vi "Launch Process.vi"(8 "error in (no error)":errorcluster, 11 "ConfigManager.Text in":refnum<class "ConfigManager.Text.lvclass">) -> (0 "error out":errorcluster, 2 "Process started":bool, 3 "ConfigManager.Text out":refnum<class "ConfigManager.Text.lvclass">)   [LabVIEW 2013, in "CfgManager.Text.lvlib" / "ConfigManager.Text.lvclass"]
uses:
  ConfigManager.Text.lvclass
  ConfigManager.Text.lvclass/ConfigManager.Text.ctl
  Process.vi
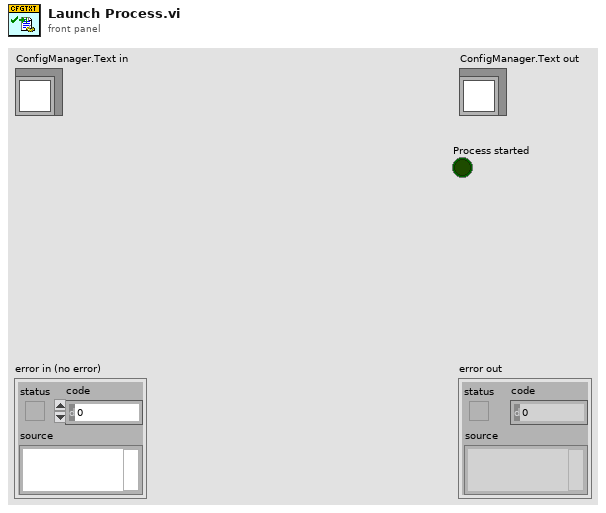
[diagram p1: front panel]
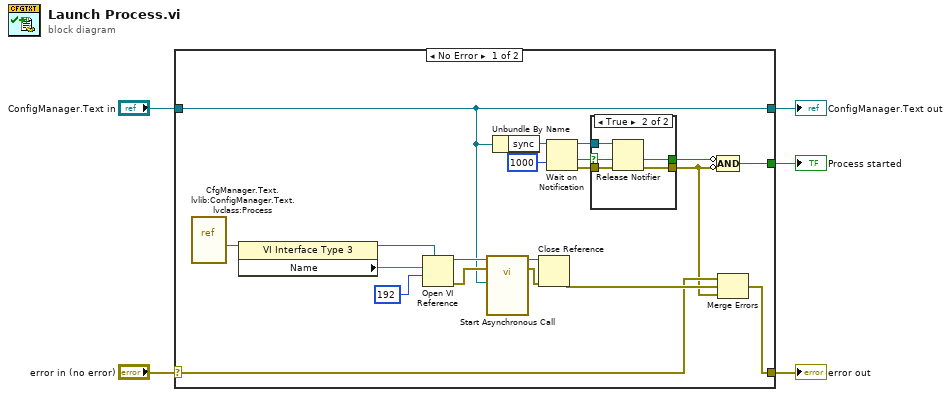
[diagram p0: block diagram]
diagram:
  n1 = case shown="No Error" "error in (no error)" {
    selector: "error in (no error)" -> [w13 w33]
    tunnel: [w12 w33] -> w4
    tunnel: [w17 w32] -> w2
    tunnel: "ConfigManager.Text in" -> [w17 w32]
    tunnel: [w11 _] -> w1
    frame No Error {
      n2 = vi-ref "CfgManager.Text.lvlib:ConfigManager.Text.lvclass:Process.vi"() -> (w25:refnum<vi>)
      n3 = property class="VI Interface Type 3"(reference=w25) -> (reference out=w19:refnum<vi>, "Name"=w18:string)  [unwired: 1 in, 1 out]
      n4 = Open VI Reference(type specifier VI Refnum (for type only)=w19, vi path=w18, options=192) -> (vi reference=w24:refnum<vi>, error out=w21:errorcluster)  [unwired: 3 in]
      n5 = call-by-ref "Start Asynchronous Call"(reference=w24, error in=w21, "ConfigManager.Text in"=w17) -> (reference out=w22:refnum<vi>, error out=w20:errorcluster)  [unwired: 9 in, 2 out]
      n6 = Unbundle By Name(w17) -> ("sync"=w16:refnum<notifier>)
      n7 = Close Reference(reference=w22, error in (no error)=w20) -> (error out=w14:errorcluster)
      n8 = Wait on Notification(notifier=w16, timeout in ms (-1)=1000) -> (notifier out=w8:refnum<notifier>, timed out?=w10:bool, error out=w9:errorcluster)  [unwired: 2 in, 1 out]
      n9 = case shown="True" w10 {
        selector: w10 -> [w26 w28]
        tunnel: w9 -> [w27 w31]
        tunnel: w8 -> [_ w30]
        tunnel: [w27 w29] -> w7
        tunnel: [w26 w28] -> w6
        frame False {
        }
        frame True {
          n10 = Release Notifier(notifier=w30, error in (no error)=w31) -> (error out=w29:errorcluster)  [unwired: 1 in, 2 out]
        }
      }
      n11 = Compound Arithmetic op=AND(invert w6, invert w7) -> (w11:bool)
      n12 = Merge Errors(w13, w14, w7) -> (w12:errorcluster)
    }
    frame Error {
    }
  }
  "error out" <- w4
  "ConfigManager.Text out" <- w2
  "Process started" <- w1
